vi "Destroy.vi"(8 "Error In":errorcluster, 11 "Display In":refnum<class "Display.lvclass">) -> (0 "Error Out":errorcluster)   [LabVIEW 2019, in "Display.lvclass"]
uses:
  Display.lvclass
  Display Element/Display Element.lvclass
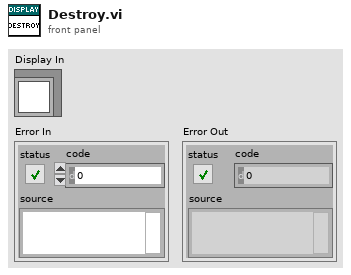
[diagram p1: front panel]
types:
  T1 = typedef "Display.lvclass/Data.ctl" = cluster{"Size":T2, "Display Elements":refnum<class "Display Element.lvclass">[], "Frame":T3}
  T2 = typedef "Display.lvclass/Size.ctl" = cluster{"Width":i32, "Length":i32}
  T3 = typedef "Display.lvclass/Frame.ctl" = cluster{"Matrix":u32[][]}
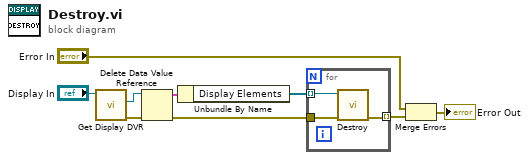
[diagram p0: block diagram]
diagram:
  n1 = call "Get Display DVR.vi"("Display In"="Display In") -> ("Error Out"=w8:errorcluster, "DVR"=w7:refnum<data-value>)  [unwired: 8 in, 1 out]
  n2 = Delete Data Value Reference(data value reference=w7, error in=w8) -> (data value=w6:T1, error out=w3:errorcluster)
  n3 = Unbundle By Name(w6) -> ("Display Elements"=w4:refnum<class "Display Element.lvclass">[])
  n4 = for {
    tunnel: w4 -> [w12] mode=indexing
    tunnel: w3 -> [w11]
    tunnel: [w10] -> w2 mode=indexing
    n5 = call-dynamic "Destroy.vi"("Error In"=w11, "Display Element In"=w12) -> ("Error Out"=w10:errorcluster)  [unwired: 9 in]
  }
  n6 = Merge Errors("Error In", w2) -> (→"Error Out":errorcluster)
